vi "extremeOfThreePixel.vi"(1 "extreme Type":u8, 2 "3":i8, 3 "2":i8, 4 "1":i8) -> (0 "extreme out":i8)   [LabVIEW 2016]
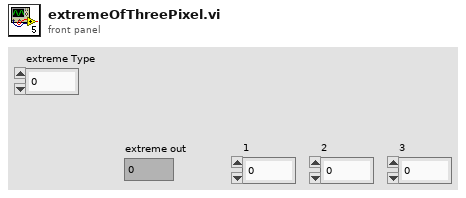
[diagram p1: front panel]
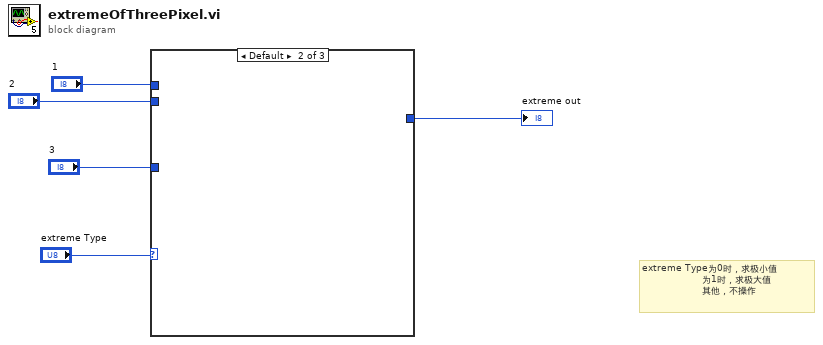
[diagram p0: block diagram]
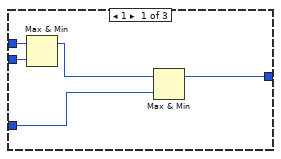
[diagram p2: hidden frame]
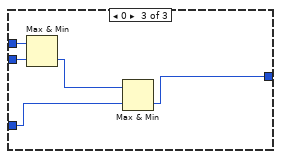
[diagram p3: hidden frame]
diagram:
  # "extreme Type为0时，求极小值\n                    为1时，求极大值\n                    其他，不操作"
  n1 = case shown="Default" "extreme Type" {
    tunnel: "1" -> [w10 _ w15]
    tunnel: "2" -> [w9 _ w14]
    tunnel: "3" -> [w7 _ w12]
    tunnel: [w6 _ w11] -> w1
    frame 1 {
      n2 = Max & Min(x=w10, y=w9) -> (max(x,y)=w8:i8)  [unwired: 1 out]
      n3 = Max & Min(x=w8, y=w7) -> (max(x,y)=w6:i8)  [unwired: 1 out]
    }
    frame Default {
    }
    frame 0 {
      n4 = Max & Min(x=w15, y=w14) -> (min(x,y)=w13:i8)  [unwired: 1 out]
      n5 = Max & Min(x=w13, y=w12) -> (min(x,y)=w11:i8)  [unwired: 1 out]
    }
  }
  "extreme out" <- w1
